vi "VLC - Process NET.vi"() -> ()   [LabVIEW 2016]
panel:
  in  "error in (no error)":errorcluster
  out "error out":errorcluster
  out "VLC Process":refnum<k24>
  in  "Script":string
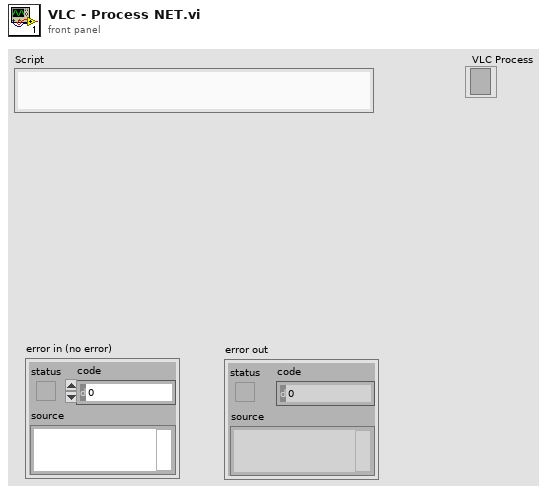
[diagram p1: front panel]
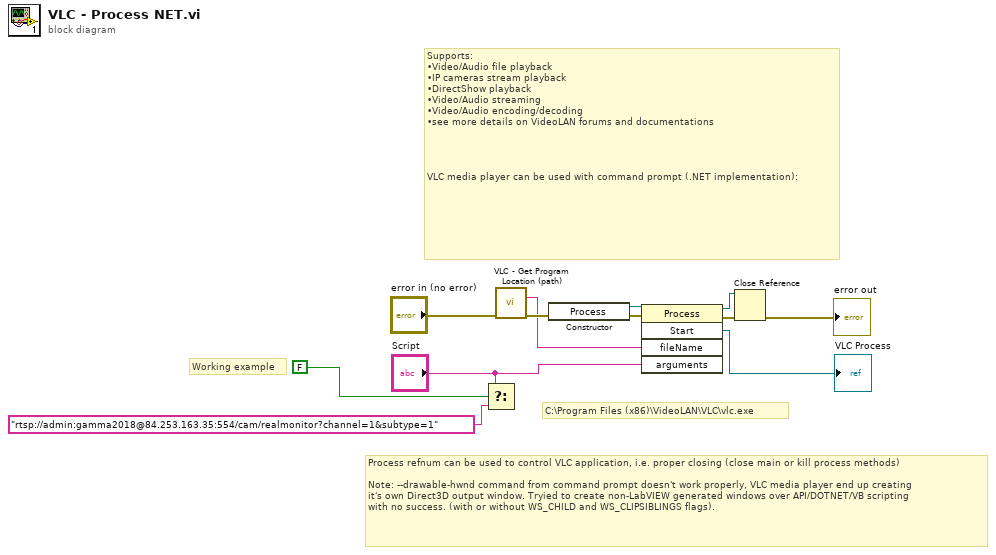
[diagram p0: block diagram]
diagram:
  # "Working example"
  # "C:\\Program Files (x86)\\VideoLAN\\VLC\\vlc.exe"
  # "Process refnum can be used to control VLC application, i.e. proper closing (close main or kill process methods)\n\nNote: --drawable-hwnd command from command prompt doesn't work properly, VLC media player end up creating \nit's own Direct3D output window. Tryied to create non-LabVIEW generated windows over API/DOTNET/VB scripting \nwith no success. (with or without WS_CHILD and WS_CLIPSIBLINGS flags)."
  # "Supports:\n•Video/Audio file playback\n•IP cameras stream playback\n•DirectShow playback\n•Video/Audio streaming\n•Video/Audio encoding/decoding\n•see more details on VideoLAN forums and documentations\n\n\n\n\nVLC media player can be used with command prompt (.NET implementation):"
  n1 = Select(t="Script", s=FALSE, f="rtsp://admin:gamma2018@84.253.163.35:554/cam/realmonitor?channel=1&subtype=1" ("Media Source")) -> ()  [unwired: 1 out]
  n2 = call "VLC - Get Program Location (path).vi"("error in (no error)"="error in (no error)") -> ("VLC path"=w8:string, "error out"=w9:errorcluster)  [unwired: 13 in]
  n3 = constructor class="Process"(error in=w9) -> (reference out=w12:refnum<k24>, error out=w11:errorcluster)  [unwired: 2 in, 1 out]
  n4 = invoke class="Process" method="Start"(reference=w12, error in=w11, "fileName"=w8, "arguments"="Script") -> (reference out=w6:refnum<k24>, error out=w7:errorcluster, "Start"=→"VLC Process":refnum<k24>)  [unwired: 1 in, 2 out]
  n5 = Close Reference(reference=w6, error in (no error)=w7) -> (error out=→"error out":errorcluster)
